vi "글로벌 1.vi"() -> ()   [LabVIEW 2018]
panel:
  in  "불리언":bool
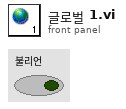
[diagram p1: front panel]
diagram:
